vi "example_llm_embedding_unit_test_1.vi"() -> ()   [LabVIEW 2020]
uses:
  src/models/message_vectors/embedding.ctl
  src/models/message_text/message_text.lvclass
  D:/Personal/LabVIEW LLMs/src/models/abstract_message_base/abstract_message_base.lvclass
  src/models/llm_openai_embedding/llm_openai_embedding.lvclass
  D:/Personal/LabVIEW LLMs/src/models/abstract_llm_base/abstract_llm_base.lvclass
  src/models/llm_gemini_embedding/llm_gemini_embedding.lvclass
  src/models/llm_ollama_embedding/llm_ollama_embedding.lvclass
  src/models/message_vectors/message_vectors.lvclass
  src/models/message_text/create_text_message.vi
  src/models/llm_openai_embedding/Instantiate_llm_openai_embed.vi
  src/models/llm_gemini_embedding/Instantiate_llm_openai_embed.vi
  src/models/llm_ollama_embedding/Instantiate_llm_ollama_embed.vi
  src/models/message_vectors/get_vector_message_value.vi
  src/models/abstract_llm_base/abstract_llm_base.lvclass
  src/utilities/env_variables/env_variables.lvlib
  src/models/abstract_llm_embedding/abstract_llm_embedding.lvclass
  D:/Personal/LabVIEW LLMs/src/models/message_vectors/message_vectors.lvclass
panel:
  in  "Provider Selector":enum32{"OpenAI", "Ollama", "Gemini"}(tab)
  in  "model_name":string(combo)="text-embedding-ada-002"
  out "openai_key":string
  in  "ollama_model_name":string(combo)="nomic-embed-text"
  in  "ollama_url":string="http://localhost:11434/"
  out "gemini_api_key":string
  in  "model_name_Gemini":string(combo)="text-embedding-004" caption="model_name"
  out "property:embedding_data":T1[](array[typedef])
  in  "Text":string[](array[string])=["Hello Pineapple", "LLM embedding is not a", "This is not a Rocket Science"]
  out "error out":errorcluster
  # "1. Ensure you assign the OpenAI Key to environmental variables so it is away from the code and easy to use the examples in future.\n\n2. Use the \"Set_ENv_Var.vi\" from examples/utils folder to set the key \"labview_llm_openai_key\"."
  # "1. Ensure you assign the OpenAI Key to environmental variables so it is away from the code and easy to use the examples in future.\n\n2. Use the \"Set_ENv_Var.vi\" from examples/utils folder to set the key \"labview_llm_gemini_key\"."
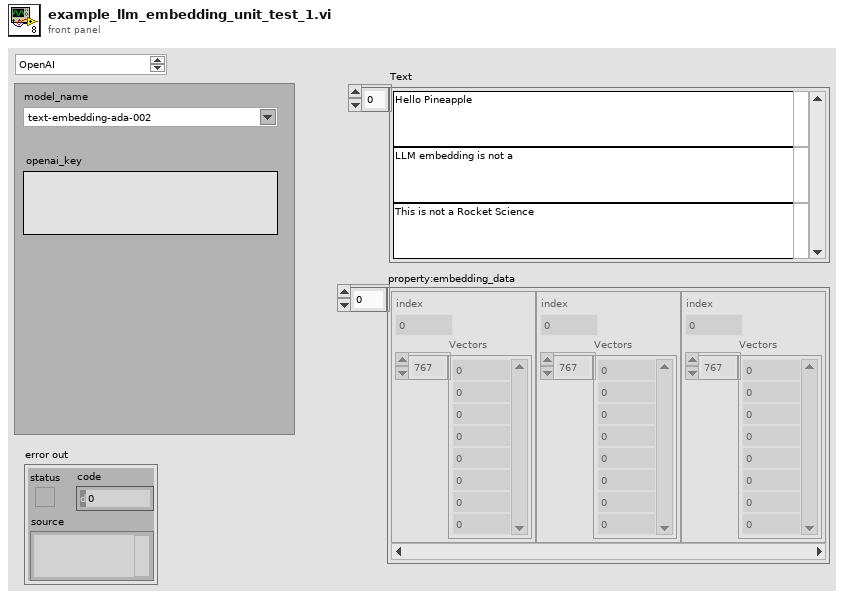
[diagram p1: front panel]
types:
  T1 = typedef "message_vectors.lvclass/embedding.ctl" = cluster{"index":u32, "Vectors":dbl[]}
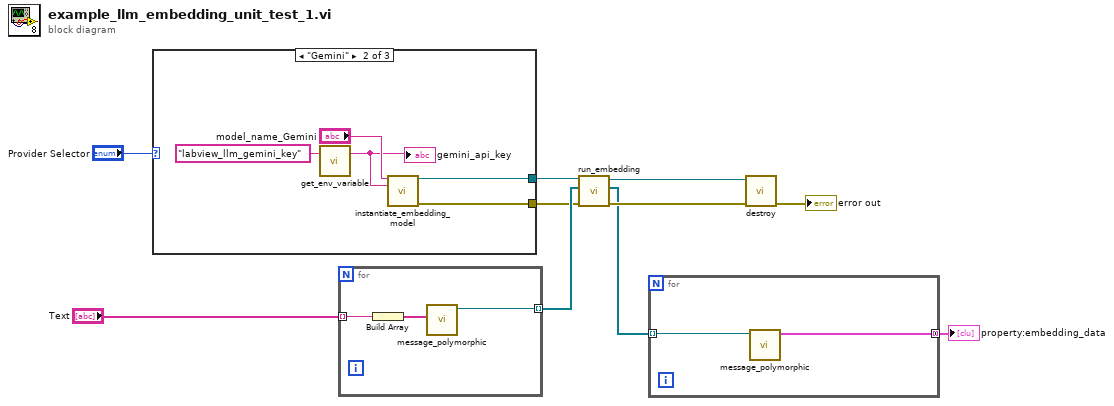
[diagram p0: block diagram]
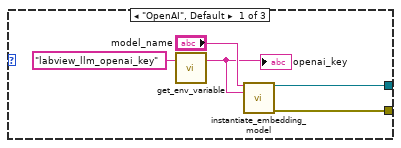
[diagram p2: hidden frame]
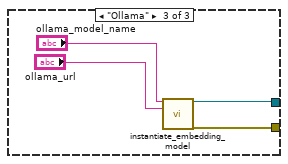
[diagram p3: hidden frame]
diagram:
  n1 = case shown="\"Gemini\"" "Provider Selector" {
    tunnel: [w14 w19 w24] -> w1
    tunnel: [w13 w18 w23] -> w3
    frame "OpenAI", Default {
      n2 = call "get_env_variable.vi"("Environment Variable Name"="labview_llm_openai_key") -> ("Value"=w11:string)  [unwired: 1 in, 1 out]
      "openai_key" <- w11
      n3 = call-poly "instantiate_embedding_model.vi"("model_name"="model_name", "openai_key"=w11) -> ("llm_openai_embedding out"=w14:refnum<class "llm_openai_embedding.lvclass">, "error out"=w13:errorcluster)  [unwired: 12 in]
    }
    frame "Gemini" {
      n4 = call "get_env_variable.vi"("Environment Variable Name"="labview_llm_gemini_key") -> ("Value"=w16:string)  [unwired: 1 in, 1 out]
      "gemini_api_key" <- w16
      n5 = call-poly "instantiate_embedding_model.vi"("model_name"="model_name_Gemini", "openai_key"=w16) -> ("llm_openai_embedding out"=w19:refnum<class "llm_gemini_embedding.lvclass">, "error out"=w18:errorcluster)  [unwired: 12 in]
    }
    frame "Ollama" {
      n6 = call-poly "instantiate_embedding_model.vi"("model_name"="ollama_model_name", "ollama_url"="ollama_url") -> ("llm_ollama_embedding out"=w24:refnum<class "llm_ollama_embedding.lvclass">, "error out"=w23:errorcluster)  [unwired: 12 in]
    }
  }
  n7 = for {
    tunnel: "Text" -> [w27] mode=indexing
    tunnel: [w26] -> w7 mode=indexing
    n8 = Build Array(w27) -> (w25:string[])
    n9 = call-poly "message_polymorphic.vi"("content"=w25) -> ("message_text out"=w26:refnum<class "message_text.lvclass">)  [unwired: 9 in, 1 out]
  }
  n10 = call "run_embedding.vi"("error in (no error)"=w3, "Messages"=w7, "abstract_llm_embedding in"=w1) -> ("error out"=w9:errorcluster, "Response"=w6:refnum<class "message_vectors.lvclass">[], "abstract_llm_embedding out"=w10:refnum<class "abstract_llm_base.lvclass">)  [unwired: 6 in]
  n11 = for {
    tunnel: [w28] -> w5 mode=concatenating
    tunnel: w6 -> [w29] mode=indexing
    n12 = call-poly "message_polymorphic.vi"("message_vectors in"=w29) -> ("embedding_data"=w28:T1[])  [unwired: 9 in, 1 out]
  }
  "property:embedding_data" <- w5
  n13 = call-dynamic "destroy.vi"("error in (no error)"=w9, "abstract_llm_base in"=w10) -> ("error out"=→"error out":errorcluster)  [unwired: 8 in, 1 out]
